vi "position.vi"(9 "枚举":enum16{"write", "read"}(ring), 11 "前面板窗口:窗口边界":T1 caption="矩形") -> (3 "前面板窗口:窗口边界 2":T1 caption="前面板窗口:窗口边界")   [LabVIEW 2018]
uses:
  <vilib>/Utility/miscctls.llb/LVRectTypeDef.ctl
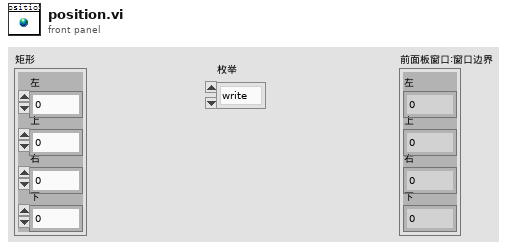
[diagram p1: front panel]
types:
  T1 = typedef "LVRectTypeDef.ctl" = cluster{"Left":i16, "Top":i16, "Right":i16, "Bottom":i16}
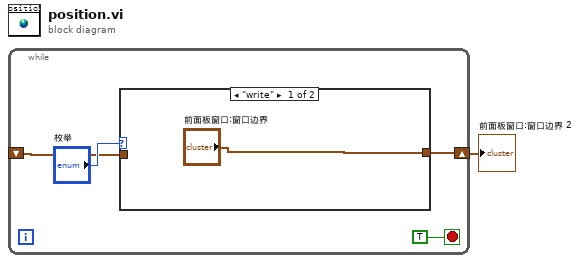
[diagram p0: block diagram]
diagram:
  n1 = while {
    shift-right: [w3] -> w1
    shift-left: _ -> [w2]
    stop <- TRUE stop-if-true
    n2 = case shown="\"write\"" "枚举" {
      tunnel: ["前面板窗口:窗口边界" w7] -> w3
      tunnel: w2 -> [_ w7]
      frame "write" {
      }
      frame "read", Default {
      }
    }
  }
  "前面板窗口:窗口边界 2" <- w1
